vi "Configure Measurement.vi"(6 "Manual Range (0)":dbl, 7 "Auto Range (T: Enable)":bool=TRUE, 8 "error in (no error)":errorcluster, 9 "Channel List(\"\")":string, 10 "Function (0: Voltage DC)":i32(ring) items=[" Voltage DC", "Voltage AC", "Current DC", "Current AC", "Resistance", "4-wire Resistance", "Diode", "Capacitance", "Temperature", "Continuity", "Frequency", "Period", "Voltage Ratio"], 11 "VISA resource name":refnum<visa-resource-name>) -> (0 "error out":errorcluster, 3 "VISA resource name out":refnum<visa-resource-name>)   [LabVIEW 2019, in "Keithley DMM6500 DAQ6500 Series.lvlib"]
doc: "Configures the measurement. Function, auto range, channel list and measure range."
uses:
  Keithley DMM6500 DAQ6500 Series.lvlib
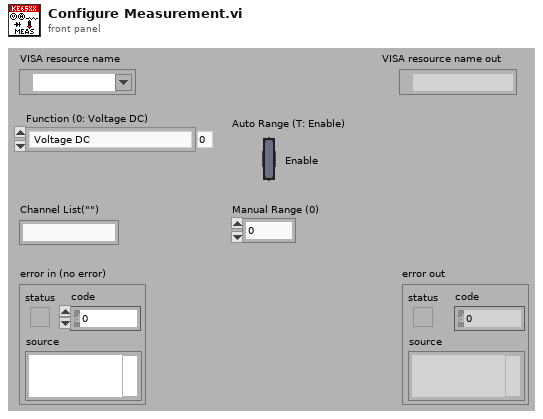
[diagram p1: front panel]
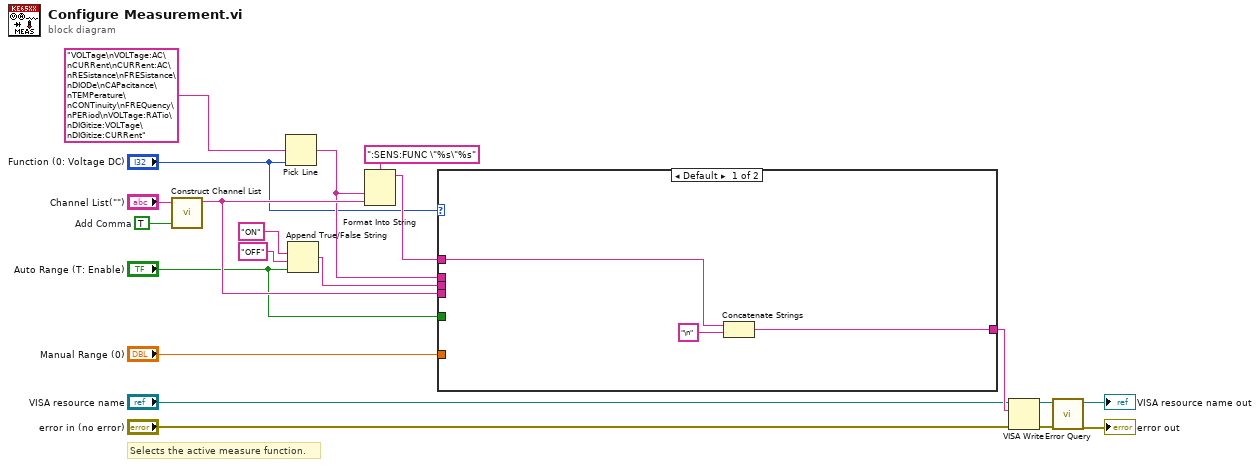
[diagram p0: block diagram]
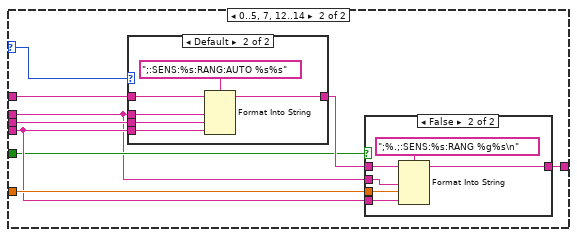
[diagram p2: hidden frame]
diagram:
  w1 = TRUE  # Add Comma
  # "Selects the active measure function."
  n1 = call "Construct Channel List.vi"("Add Comma (True)"=w1, "Channel List"="Channel List(\"\")") -> ("Channel List String"=w6:string)  [unwired: 1 in]
  n2 = Pick Line(multi-line string="VOLTage\nVOLTage:AC\nCURRent\nCURRent:AC\nRESistance\nFRESistance\nDIODe\nCAPacitance\nTEMPerature\nCONTinuity\nFREQuency\nPERiod\nVOLTage:RATio\nDIGitize:VOLTage\nDIGitize:CURRent", line index="Function (0: Voltage DC)") -> (output string=w3:string)  [unwired: 1 in]
  n3 = Append True/False String(1:"Auto Range (T: Enable)", 2:"OFF", 3:"ON") -> (0:w16:string)  [unwired: 1 in]
  n4 = Format Into String(format string=":SENS:FUNC \"%s\"%s", w3, w6) -> (resulting string=w17:string)  [unwired: 2 in, 1 out]
  n5 = case shown="Default" "Function (0: Voltage DC)" {
    selector: "Function (0: Voltage DC)" -> [_ w24]
    tunnel: w17 -> [w22 w32]
    tunnel: w16 -> [_ w31]
    tunnel: "Manual Range (0)" -> [_ w29]
    tunnel: [w21 w28] -> w14
    tunnel: w6 -> [_ w27]
    tunnel: "Auto Range (T: Enable)" -> [_ w26]
    tunnel: w3 -> [_ w25]
    frame Default {
      n6 = Concatenate Strings(w22, "\n") -> (w21:string)
    }
    frame 0..5, 7, 12..14 {
      n7 = case shown="Default" w24 {
        tunnel: w32 -> [w33 w39]
        tunnel: w31 -> [_ w37]
        tunnel: [w33 w36] -> w30
        tunnel: w27 -> [_ w35]
        tunnel: w25 -> [_ w34]
        frame 14, 15 {
        }
        frame Default {
          n8 = Format Into String(format string=";:SENS:%s:RANG:AUTO %s%s", initial string=w39, w34, w37, w35) -> (resulting string=w36:string)  [unwired: 1 in, 1 out]
        }
      }
      n9 = case shown="False" w26 {
        tunnel: w30 -> [w40 w46]
        tunnel: w29 -> [_ w44]
        tunnel: [w40 w43] -> w28
        tunnel: w27 -> [_ w42]
        tunnel: w25 -> [_ w41]
        frame True {
        }
        frame False {
          n10 = Format Into String(format string=";%.;:SENS:%s:RANG %g%s\n", initial string=w46, w41, w44, w42) -> (resulting string=w43:string)  [unwired: 1 in, 1 out]
        }
      }
    }
  }
  n11 = VISA Write(VISA resource name="VISA resource name", write buffer=w14, error in (no error)="error in (no error)") -> (VISA resource name out=w11:refnum<visa-resource-name>, error out=w10:errorcluster)  [unwired: 1 out]
  n12 = call "Error Query.vi"("error in (no error)"=w10, "VISA resource name"=w11) -> ("error out"=→"error out":errorcluster, "VISA resource name out"=→"VISA resource name out":refnum<visa-resource-name>)  [unwired: 6 in, 2 out]
